vi "StartCamera.vi"(11 "WebCamViewerRef":refnum<k24>) -> (3 "GetCameras":string[](array[string]))   [LabVIEW 2020]
uses:
  D:/LabviewDXFViewer/LabviewDXFViewer/bin/Release/LabviewDXFViewer.exe
  LabviewDXFViewer/bin/Release/LabviewDXFViewer.exe
panel:
  out "error out":errorcluster
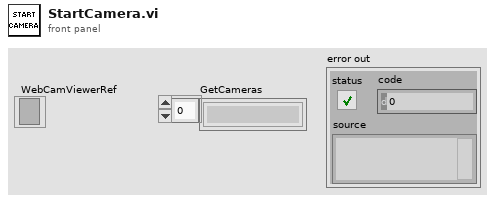
[diagram p1: front panel]
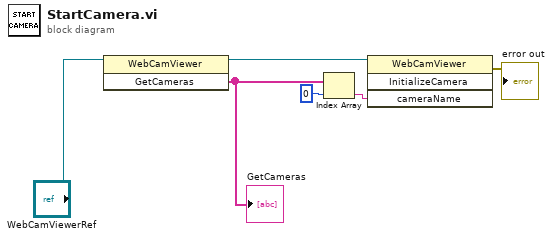
[diagram p0: block diagram]
diagram:
  n1 = invoke class="WebCamViewer" method="GetCameras"(reference="WebCamViewerRef") -> (reference out=w2:refnum<k24>, "GetCameras"=w4:string[])  [unwired: 2 in, 1 out]
  "GetCameras" <- w4
  n2 = Index Array(array=w4, index=0) -> (element=w3:string)
  n3 = invoke class="WebCamViewer" method="InitializeCamera"(reference=w2, "cameraName"=w3) -> (error out=→"error out":errorcluster)  [unwired: 2 in, 3 out]
